vi "Ping_toArduino.vi"(8 "error in (no error)":errorcluster, 11 "VISA Refnum in":refnum<visa-resource-name>) -> (0 "error out":errorcluster, 2 "PING OK":bool, 3 "VISA Refnum out":refnum<visa-resource-name>)   [LabVIEW 2019, in "SHARED VI'S.lvlib"]
uses:
  SHARED VI'S.lvlib
  <vilib>/Utility/error.llb/Error Cluster From Error Code.vi
  <vilib>/ErrorRing/Error Ring.xnode
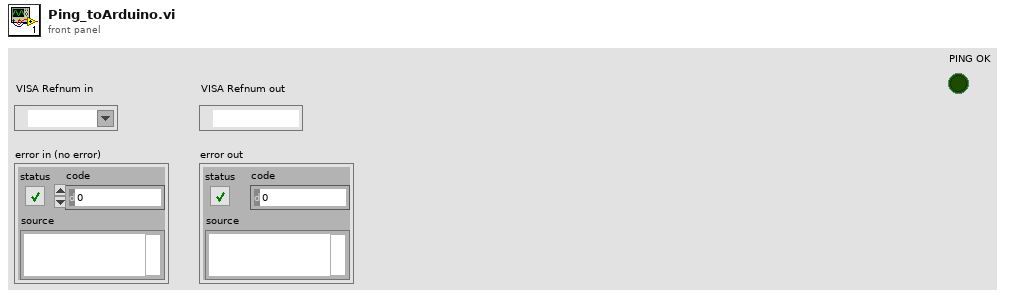
[diagram p1: front panel]
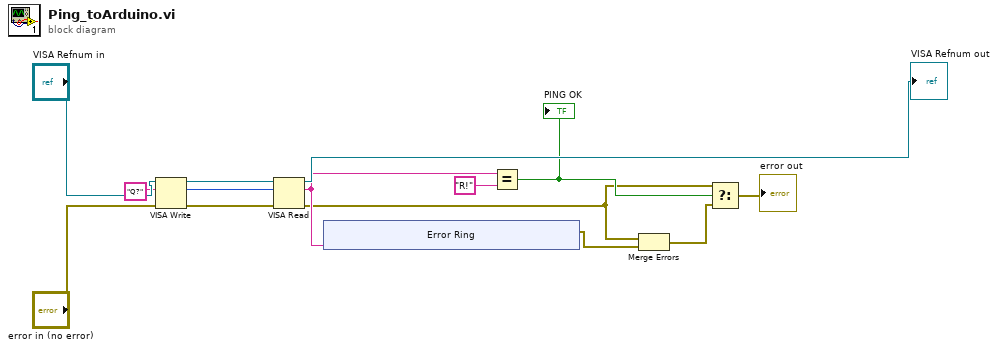
[diagram p0: block diagram]
diagram:
  n1 = VISA Write(VISA resource name="VISA Refnum in", write buffer="Q?", error in (no error)="error in (no error)") -> (VISA resource name out=w13:refnum<visa-resource-name>, return count=w7:u32, error out=w8:errorcluster)
  n2 = VISA Read(VISA resource name=w13, byte count=w7, error in (no error)=w8) -> (VISA resource name out=→"VISA Refnum out":refnum<visa-resource-name>, read buffer=w10:string, error out=w2:errorcluster)  [unwired: 1 out]
  n3 = xnode "Error Ring"("parameter 0"=w10) -> ("error out"=w4:errorcluster)
  n4 = Equal?(x=w10, y="R!") -> (x = y?=w5:bool)
  "PING OK" <- w5
  n5 = Merge Errors(w2, w4) -> (w3:errorcluster)
  n6 = Select(t=w2, s=w5, f=w3) -> (s? t:f=→"error out":errorcluster)
